vi "一台设备.vi"() -> ()   [LabVIEW 2012]
uses:
  <vilib>/Analysis/NI_AALPro.lvlib
panel:
  in  "?":enum32{"振动", "FFT", "转速", "温度湿度"}(tab)
  out "?":i16[](graph)
  out "?":i16[](graph)
  out "?":i16[](graph)
  out "?":i16[](graph)
  out "?":dbl[](graph)
  out "?":dbl[](graph)
  out "?":dbl[](graph)
  out "?":dbl[](graph)
  out "?":u16[](graph)
  out "?":dbl(graph)
  out "?":dbl(graph)
  out "?":dbl(graph)
  out "?":dbl(graph)
  out "?":dbl(graph)
  out "?":dbl(graph)
  out "?":u8(graph)
  out "?":u8(graph)
  out "系统时间":string
  out "收包":i32
  out "KB/s":dbl
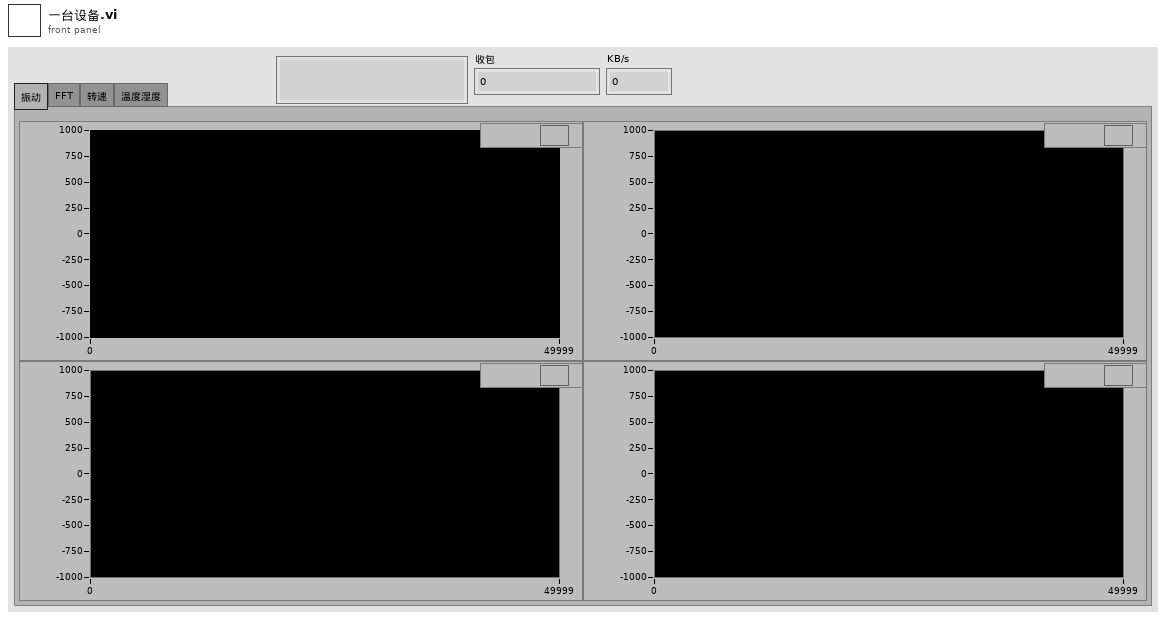
[diagram p1: front panel]
types:
  T1 = enum16{"open", "replace", "create", "open or create", "replace or create", "replace or create with confirmation"}
  T2 = enum16{"big-endian, network order", "native, host order", "little-endian"}
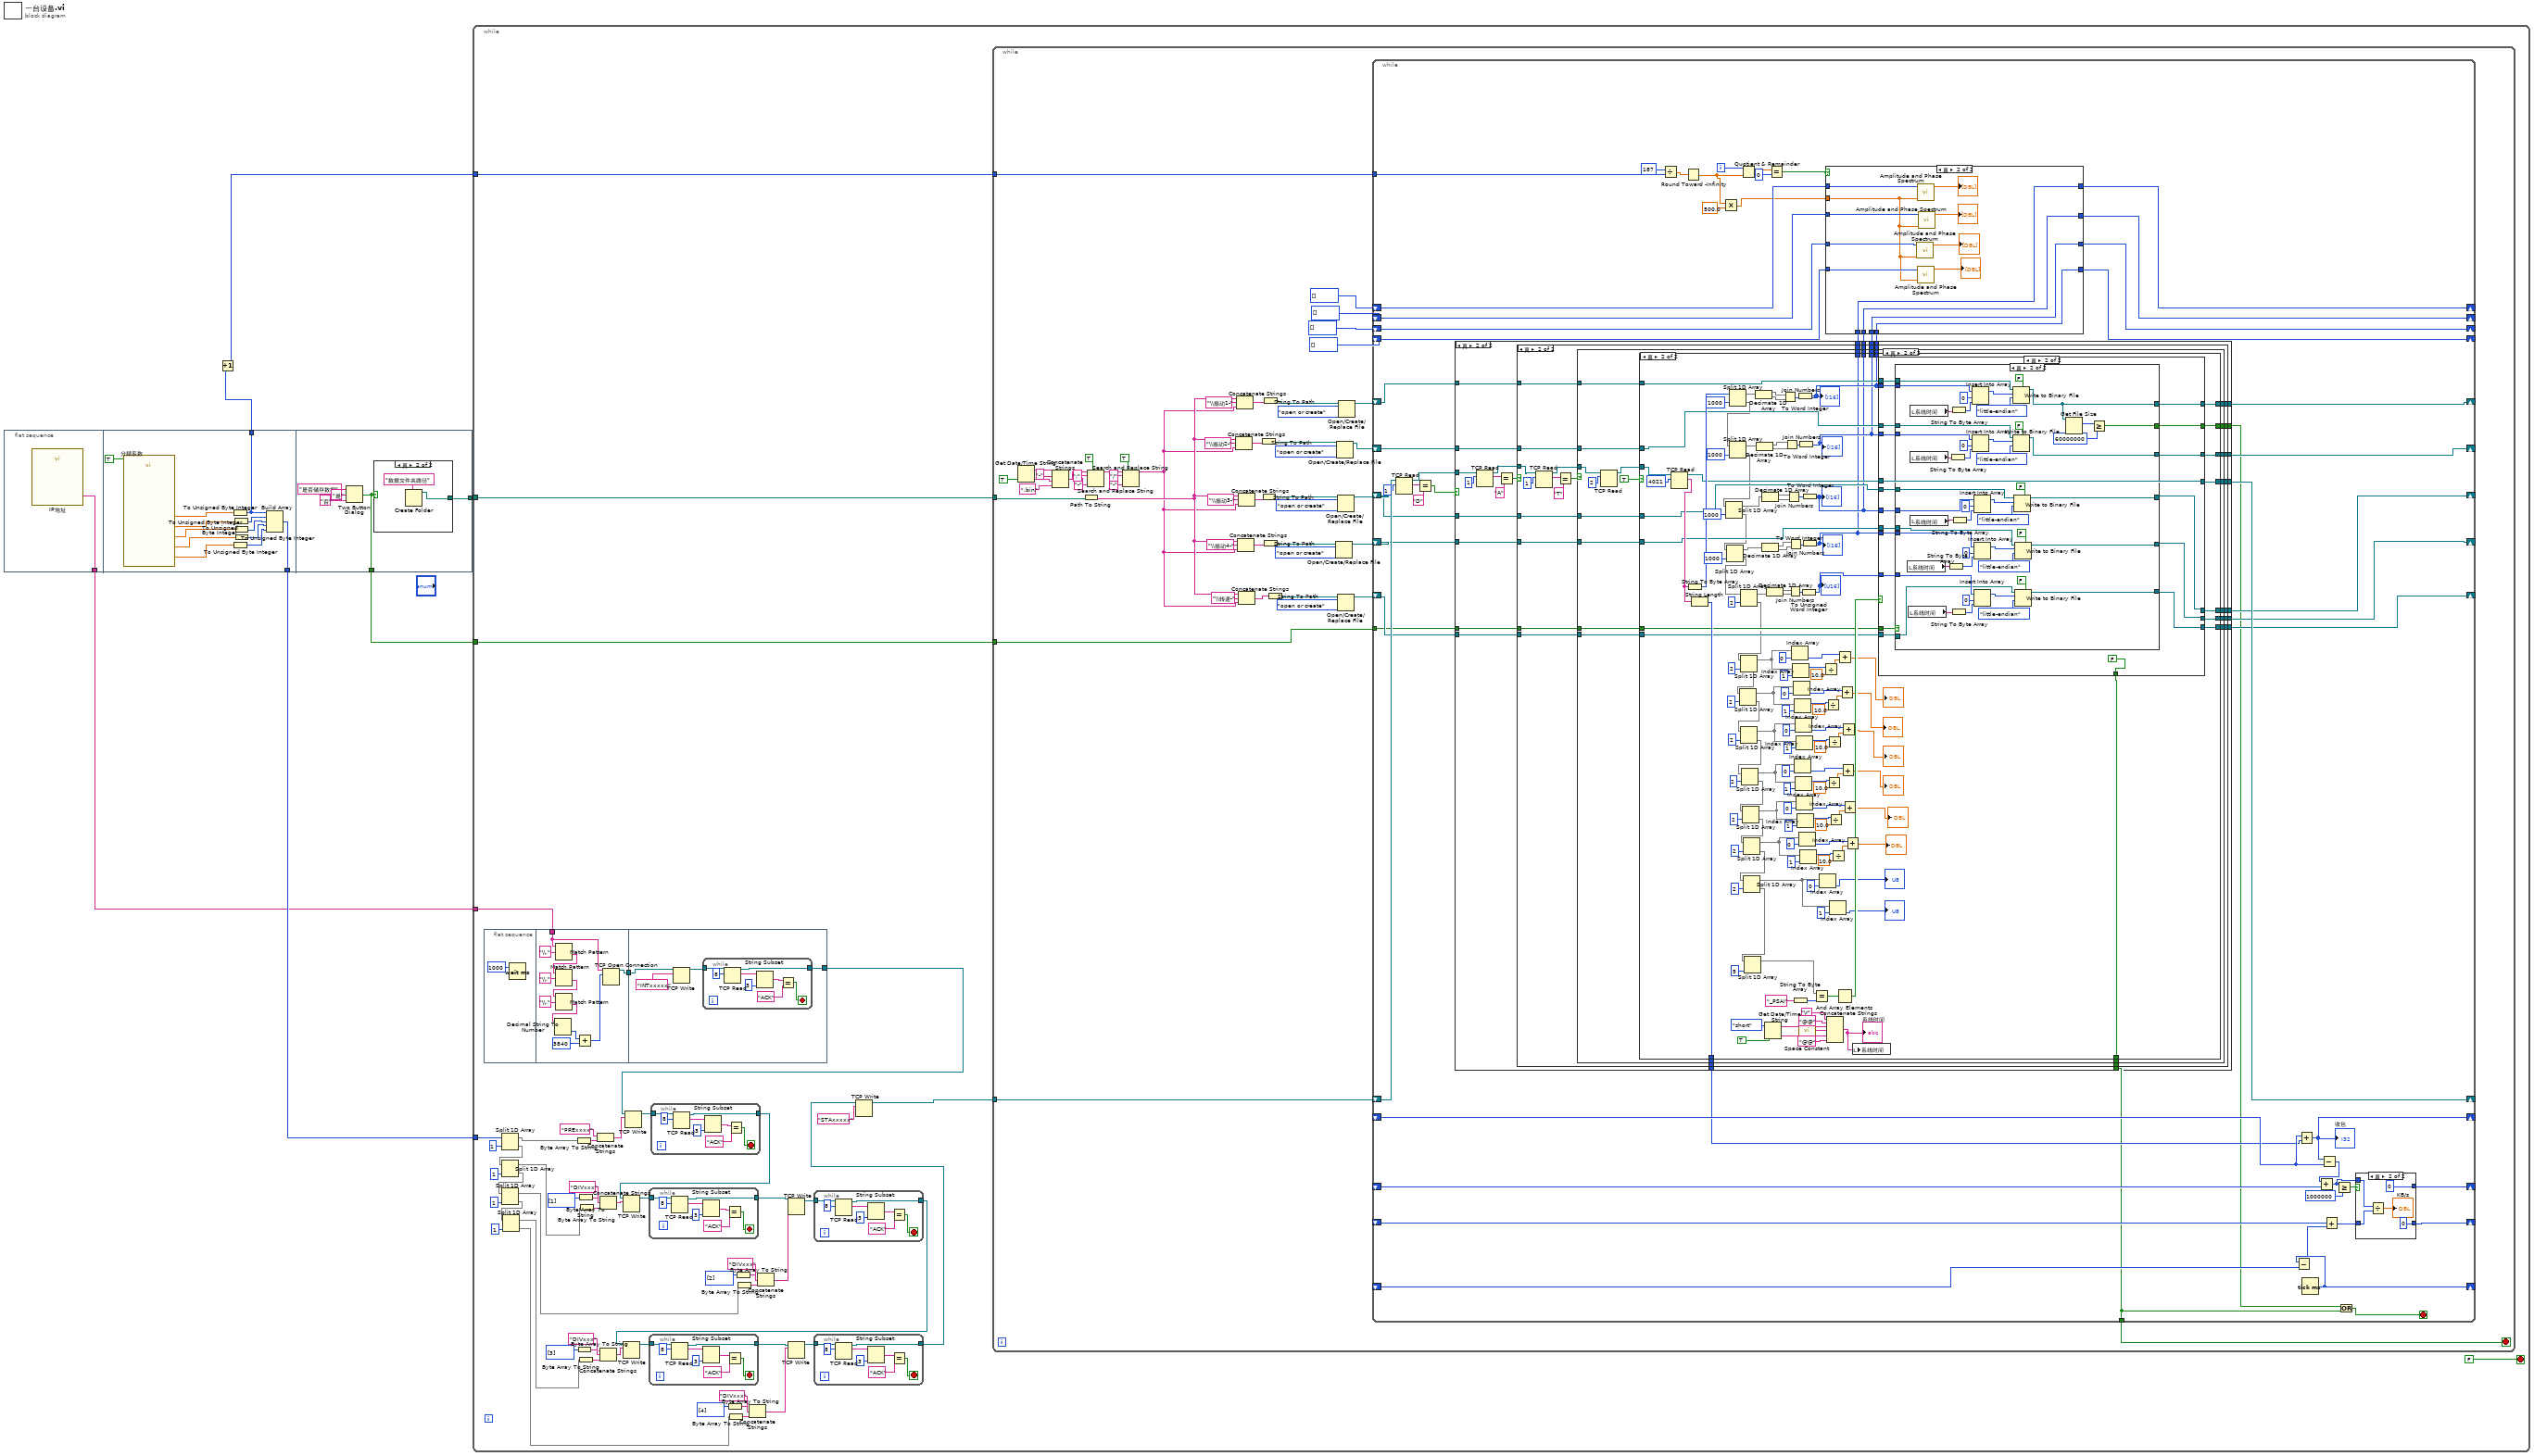
[diagram p0: block diagram]
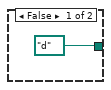
[diagram p2: hidden frame]
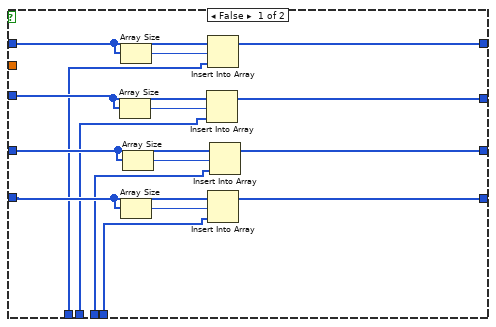
[diagram p3: hidden frame]
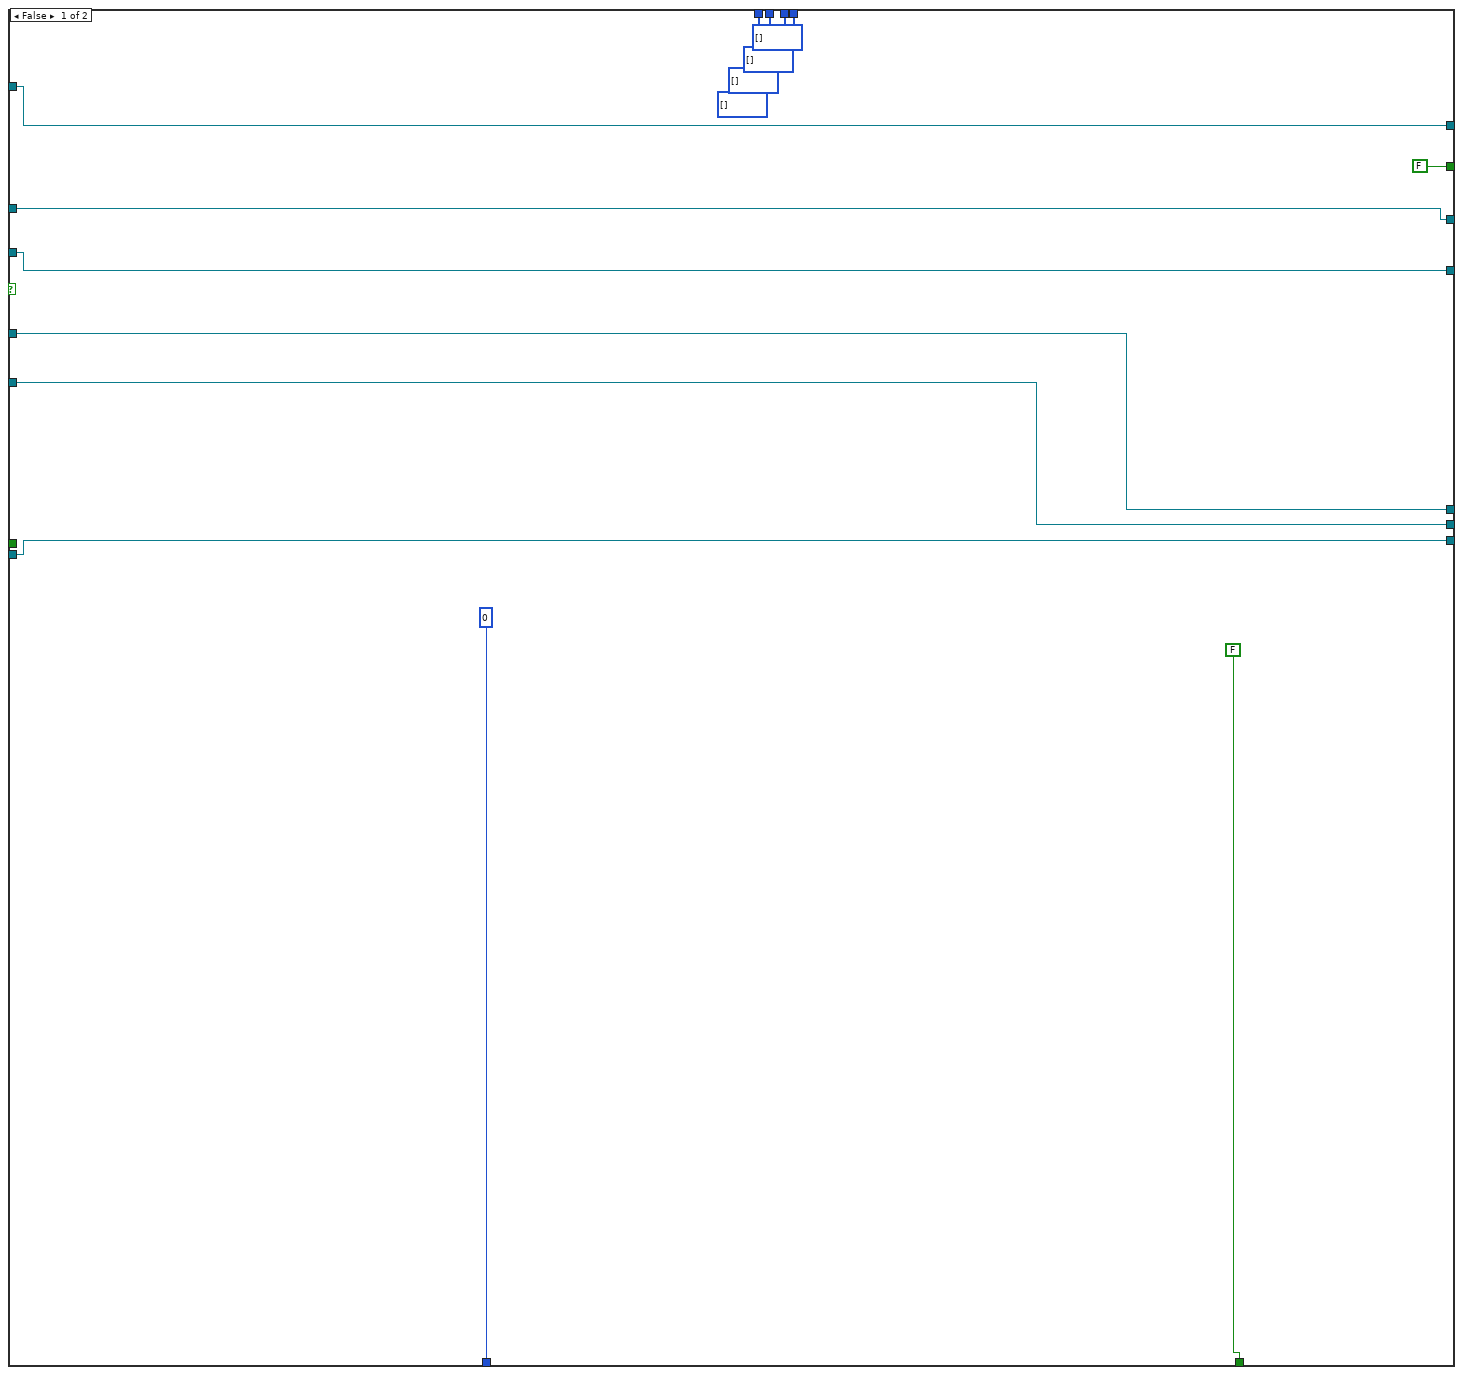
[diagram p4: hidden frame]
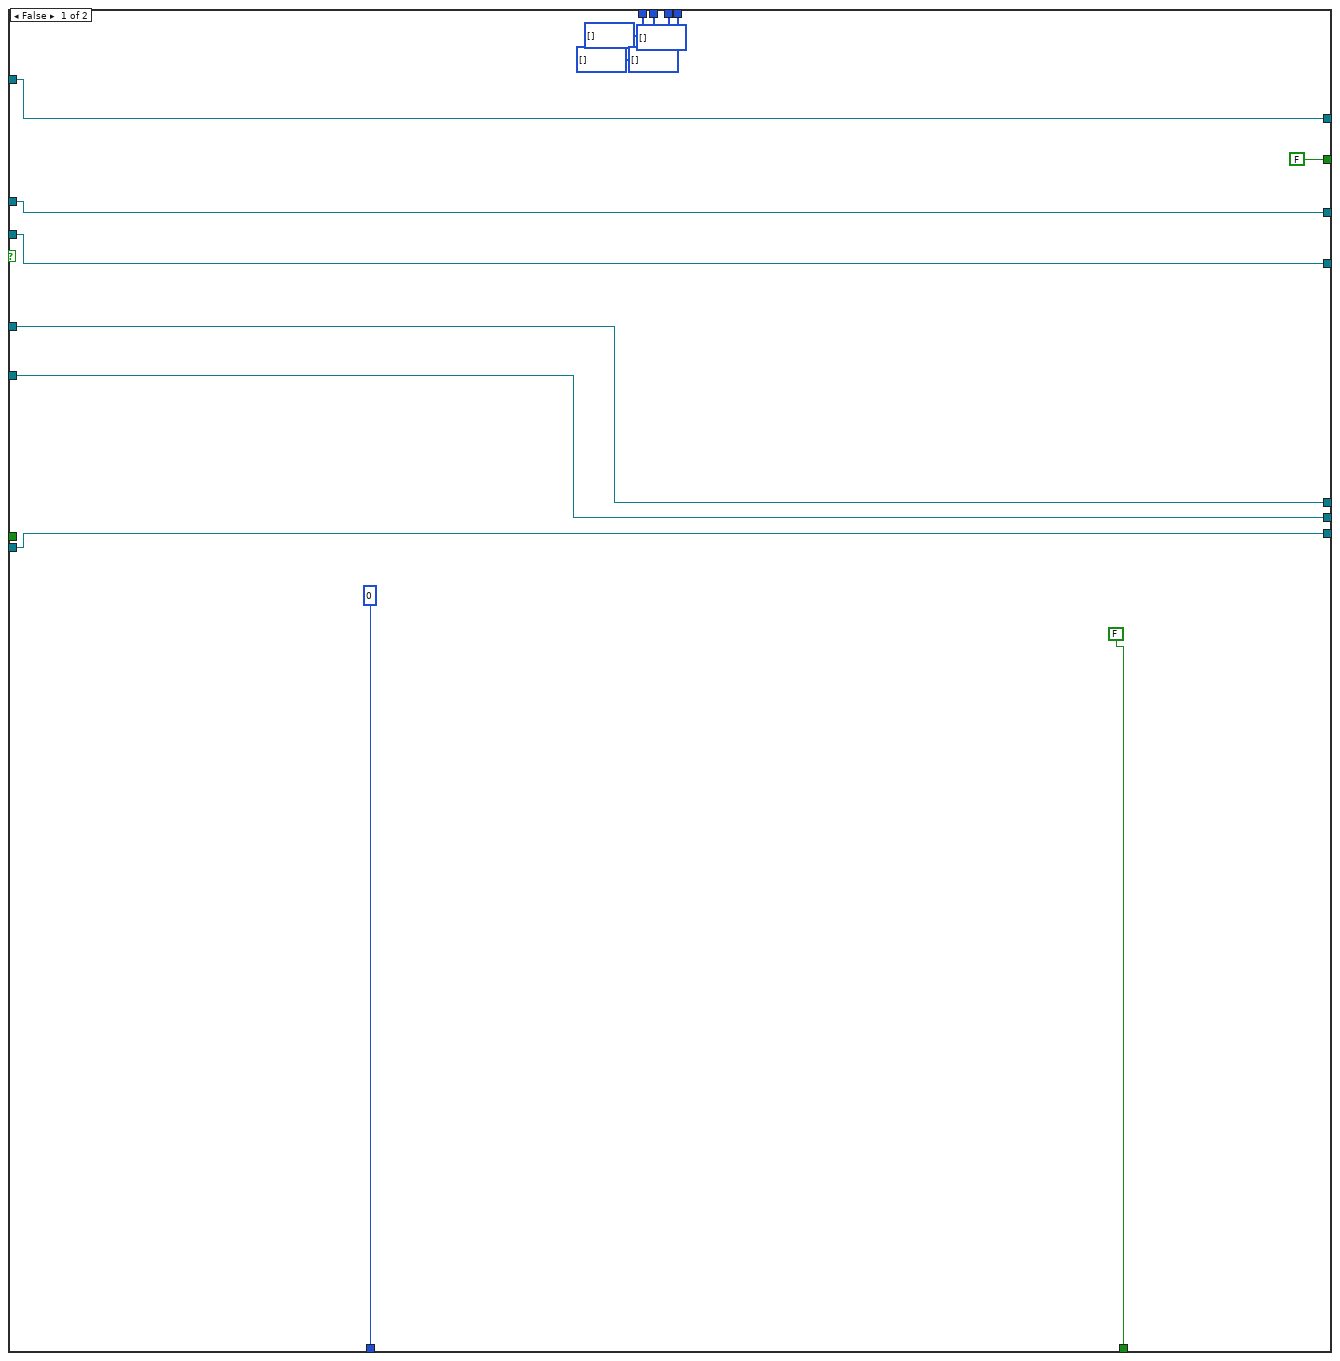
[diagram p5: hidden frame]
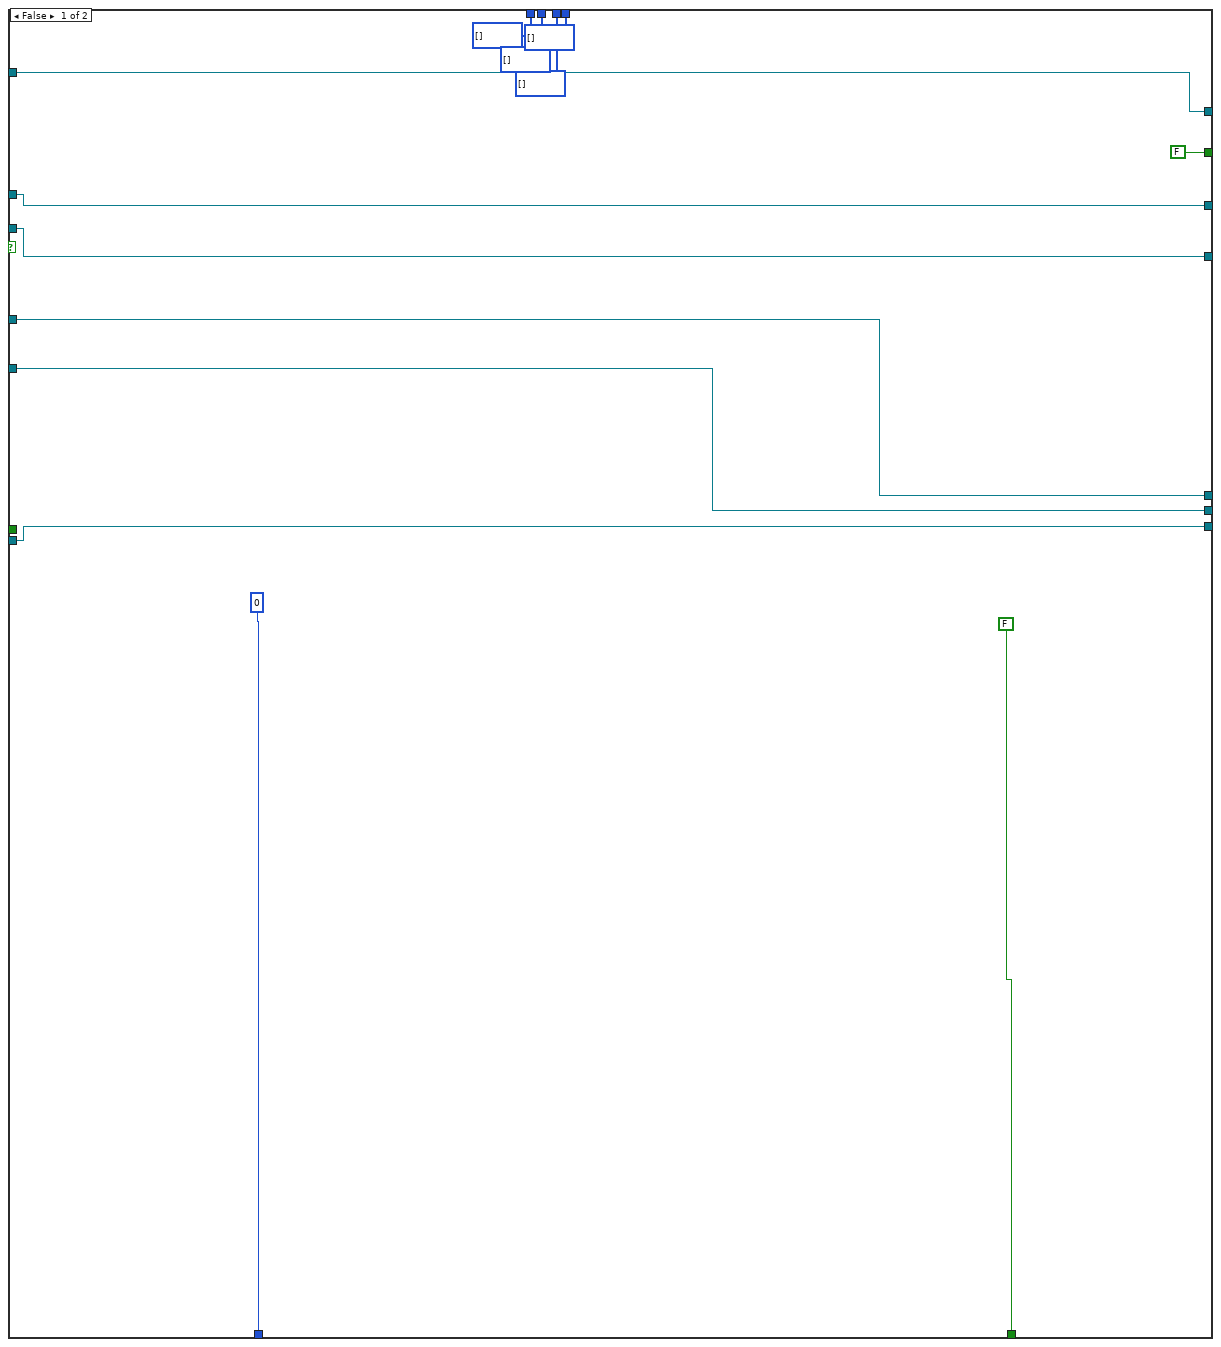
[diagram p6: hidden frame]
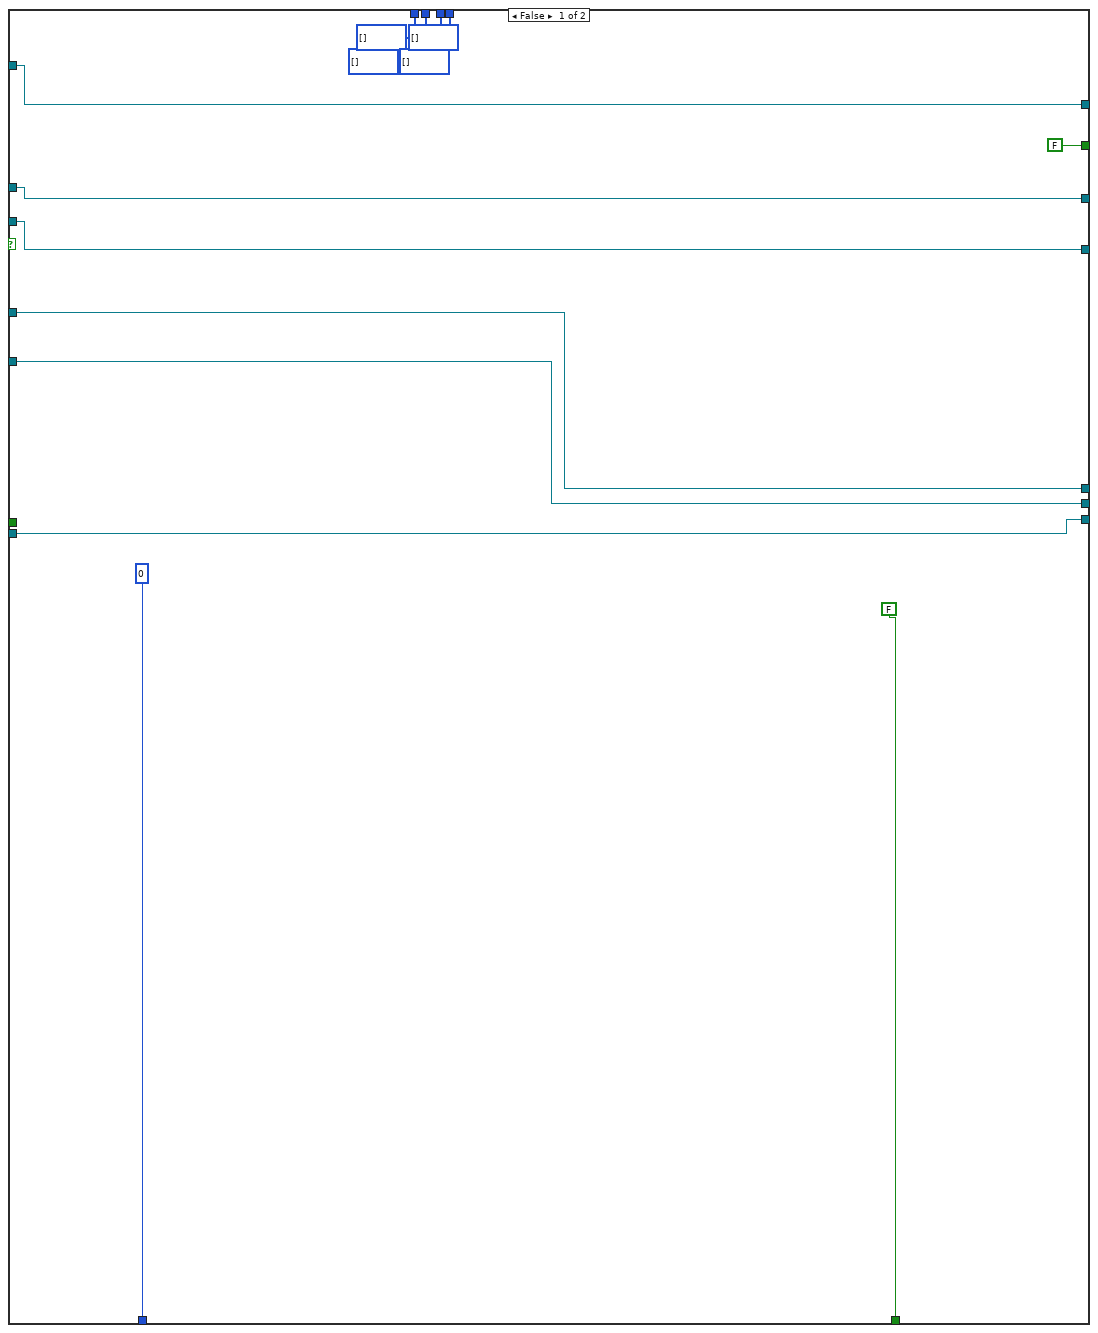
[diagram p7: hidden frame]
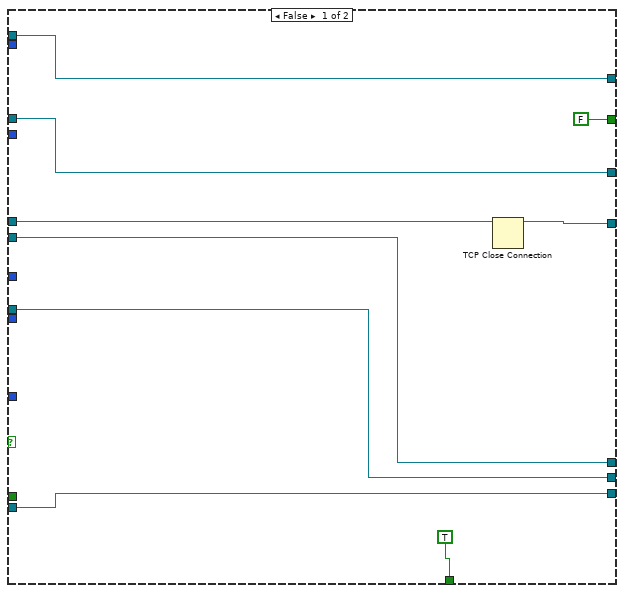
[diagram p8: hidden frame]
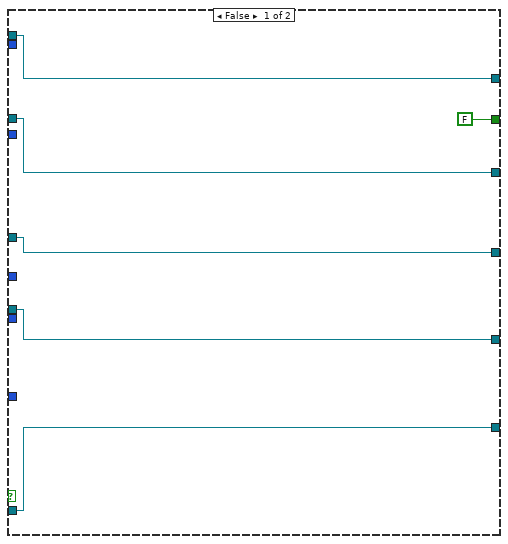
[diagram p9: hidden frame]
diagram:
  n1 = flat-sequence {
    tunnel: [w7] -> w1
    tunnel: [w14] -> w4
    tunnel: [w8] -> w3
    tunnel: [w21] -> w5
    tunnel: [w20] -> w6
    frame #0 {
      n2 = call "IP地址"() -> ("IP地址"=w7:string)  [unwired: 17 in, 2 out]
    }
    frame #1 {
      n3 = call "分频系数"("Enable"=TRUE) -> ("#4分频系数"=w12:dbl, "#3分频系数"=w11:dbl, "#2分频系数"=w10:dbl, "#1分频系数"=w9:dbl, "总分频系数"=w13:dbl)  [unwired: 12 in, 2 out]
      n4 = To Unsigned Byte Integer(number=w13) -> (unsigned 8bit integer=w8:u8)
      n5 = To Unsigned Byte Integer(number=w12) -> (unsigned 8bit integer=w15:u8)
      n6 = To Unsigned Byte Integer(number=w9) -> (unsigned 8bit integer=w18:u8)
      n7 = To Unsigned Byte Integer(number=w10) -> (unsigned 8bit integer=w17:u8)
      n8 = To Unsigned Byte Integer(number=w11) -> (unsigned 8bit integer=w16:u8)
      n9 = Build Array(w8, w18, w17, w16, w15) -> (w14:u8[])
    }
    frame #2 {
      n10 = Two Button Dialog(message="是否储存数据" ("消息"), 1:"否" ("F按钮名称（“取消”）"), 2:"是" ("T按钮名称（“确定”）")) -> (T button?=w20:bool)
      n11 = case shown="真" w20 {
        tunnel: [path "d:/" ("路径（使用对话框）") w27] -> w21
        frame False {
        }
        frame True {
          n12 = Create Folder(prompt (Create Folder)="数据文件夹路径" ("对话框窗口（创建文件夹）")) -> (created path=w27:path)  [unwired: 2 in, 2 out]
        }
      }
    }
  }
  n13 = Increment(x=w3) -> (x+1=w2:u8)
  n14 = while {
    tunnel: w6 -> [w81]
    tunnel: w5 -> [w80]
    tunnel: w4 -> [w66]
    tunnel: w2 -> [w79]
    tunnel: w1 -> [w28]
    stop <- FALSE stop-if-true
    n15 = flat-sequence {
      tunnel: [w94] -> w30
      tunnel: w28 -> [w85]
      tunnel: w30 -> [w97]
      tunnel: [w95] -> w29
      frame #0 {
        n16 = Wait (ms)(milliseconds to wait=u32 1000 ("毫秒倍数")) -> ()  [unwired: 1 out]
      }
      frame #1 {
        n17 = Match Pattern(string=w85, regular expression="\\." ("正则表达式")) -> (after substring=w89:string)  [unwired: 1 in, 3 out]
        n18 = Match Pattern(string=w89, regular expression="\\." ("正则表达式")) -> (after substring=w90:string)  [unwired: 1 in, 3 out]
        n19 = Match Pattern(string=w90, regular expression="\\." ("正则表达式")) -> (after substring=w91:string)  [unwired: 1 in, 3 out]
        n20 = Decimal String To Number(string=w91) -> (number=w92:i32)  [unwired: 2 in, 1 out]
        n21 = Add(x=w92, y=3840) -> (x+y=w84:i32)
        n22 = TCP Open Connection(address=w85, remote port or service name=w84) -> (connection ID=w94:refnum<k5>)  [unwired: 3 in, 1 out]
      }
      frame #2 {
        n23 = TCP Write(connection ID=w97, data in="INTxxxxx" ("数据输入")) -> (connection ID out=w96:refnum<k5>)  [unwired: 2 in, 2 out]
        n24 = while {
          tunnel: w96 -> [w106]
          tunnel: [w100] -> w95
          stop <- w101 stop-if-true
          n25 = TCP Read(connection ID=w106, bytes to read=8 ("读取的字节")) -> (connection ID out=w100:refnum<k5>, data out=w104:string)  [unwired: 3 in, 1 out]
          n26 = String Subset(string=w104, length (rest)=3 ("偏移量(0)")) -> (substring=w103:string)  [unwired: 1 in]
          n27 = Equal?(x=w103, y="ACK") -> (x = y?=w101:bool)
        }
      }
    }
    n28 = Split 1D Array(array=w66, index=1 ("索引")) -> (first subarray=w64:u8[], second subarray=w60:u8[])
    n29 = Split 1D Array(array=w60, index=1 ("索引")) -> (first subarray=w40:u8[], second subarray=w59:u8[])
    n30 = Split 1D Array(array=w59, index=1 ("索引")) -> (first subarray=w39:u8[], second subarray=w58:u8[])
    n31 = Split 1D Array(array=w58, index=1 ("索引")) -> (first subarray=w38:u8[], second subarray=w37:u8[])
    n32 = Byte Array To String(unsigned byte array=w64) -> (string=w69:string)
    n33 = Byte Array To String(unsigned byte array=u8[] [3] ("无符号字节数组")) -> (string=w46:string)
    n34 = Byte Array To String(unsigned byte array=u8[] [1] ("无符号字节数组")) -> (string=w54:string)
    n35 = Byte Array To String(unsigned byte array=w38) -> (string=w48:string)
    n36 = Byte Array To String(unsigned byte array=w40) -> (string=w57:string)
    n37 = Concatenate Strings("PRExxxx" ("数据输入"), w69) -> (w67:string)
    n38 = Concatenate Strings("DIVxxx" ("数据输入"), w54, w57) -> (w56:string)
    n39 = Concatenate Strings("DIVxxx" ("数据输入"), w46, w48) -> (w31:string)
    n40 = TCP Write(connection ID=w29, data in=w67) -> (connection ID out=w78:refnum<k5>)  [unwired: 2 in, 2 out]
    n41 = while {
      tunnel: w78 -> [w146]
      tunnel: [w140] -> w73
      stop <- w141 stop-if-true
      n42 = TCP Read(connection ID=w146, bytes to read=8 ("读取的字节")) -> (connection ID out=w140:refnum<k5>, data out=w144:string)  [unwired: 3 in, 1 out]
      n43 = String Subset(string=w144, length (rest)=3 ("偏移量(0)")) -> (substring=w143:string)  [unwired: 1 in]
      n44 = Equal?(x=w143, y="ACK") -> (x = y?=w141:bool)
    }
    n45 = TCP Write(connection ID=w73, data in=w56) -> (connection ID out=w77:refnum<k5>)  [unwired: 2 in, 2 out]
    n46 = while {
      tunnel: w77 -> [w138]
      tunnel: [w132] -> w72
      stop <- w133 stop-if-true
      n47 = TCP Read(connection ID=w138, bytes to read=8 ("读取的字节")) -> (connection ID out=w132:refnum<k5>, data out=w136:string)  [unwired: 3 in, 1 out]
      n48 = String Subset(string=w136, length (rest)=3 ("偏移量(0)")) -> (substring=w135:string)  [unwired: 1 in]
      n49 = Equal?(x=w135, y="ACK") -> (x = y?=w133:bool)
    }
    n50 = Byte Array To String(unsigned byte array=u8[] [4] ("无符号字节数组")) -> (string=w42:string)
    n51 = Byte Array To String(unsigned byte array=w37) -> (string=w44:string)
    n52 = Byte Array To String(unsigned byte array=u8[] [2] ("无符号字节数组")) -> (string=w50:string)
    n53 = Byte Array To String(unsigned byte array=w39) -> (string=w52:string)
    n54 = Concatenate Strings("DIVxxx" ("数据输入"), w42, w44) -> (w35:string)
    n55 = Concatenate Strings("DIVxxx" ("数据输入"), w50, w52) -> (w36:string)
    n56 = TCP Write(connection ID=w72, data in=w36) -> (connection ID out=w76:refnum<k5>)  [unwired: 2 in, 2 out]
    n57 = while {
      tunnel: w76 -> [w130]
      tunnel: [w124] -> w71
      stop <- w125 stop-if-true
      n58 = TCP Read(connection ID=w130, bytes to read=8 ("读取的字节")) -> (connection ID out=w124:refnum<k5>, data out=w128:string)  [unwired: 3 in, 1 out]
      n59 = String Subset(string=w128, length (rest)=3 ("偏移量(0)")) -> (substring=w127:string)  [unwired: 1 in]
      n60 = Equal?(x=w127, y="ACK") -> (x = y?=w125:bool)
    }
    n61 = TCP Write(connection ID=w71, data in=w31) -> (connection ID out=w75:refnum<k5>)  [unwired: 2 in, 2 out]
    n62 = while {
      tunnel: w75 -> [w122]
      tunnel: [w116] -> w70
      stop <- w117 stop-if-true
      n63 = TCP Read(connection ID=w122, bytes to read=8 ("读取的字节")) -> (connection ID out=w116:refnum<k5>, data out=w120:string)  [unwired: 3 in, 1 out]
      n64 = String Subset(string=w120, length (rest)=3 ("偏移量(0)")) -> (substring=w119:string)  [unwired: 1 in]
      n65 = Equal?(x=w119, y="ACK") -> (x = y?=w117:bool)
    }
    n66 = TCP Write(connection ID=w70, data in=w35) -> (connection ID out=w74:refnum<k5>)  [unwired: 2 in, 2 out]
    n67 = while {
      tunnel: w74 -> [w114]
      tunnel: [w108] -> w34
      stop <- w109 stop-if-true
      n68 = TCP Read(connection ID=w114, bytes to read=8 ("读取的字节")) -> (connection ID out=w108:refnum<k5>, data out=w112:string)  [unwired: 3 in, 1 out]
      n69 = String Subset(string=w112, length (rest)=3 ("偏移量(0)")) -> (substring=w111:string)  [unwired: 1 in]
      n70 = Equal?(x=w111, y="ACK") -> (x = y?=w109:bool)
    }
    n71 = TCP Write(connection ID=w34, data in="STAxxxxx" ("数据输入")) -> (connection ID out=w32:refnum<k5>)  [unwired: 2 in, 2 out]
    n72 = while {
      tunnel: w32 -> [w195]
      tunnel: w81 -> [w194]
      tunnel: w80 -> [w167]
      tunnel: w79 -> [w147]
      stop <- w157 stop-if-true
      n73 = Get Date/Time String(want seconds? (F)=TRUE ("需要秒？(F)")) -> (date string=w165:string, time string=w162:string)  [unwired: 2 in]
      n74 = Concatenate Strings(w165, "-" ("字符串"), w162, ".bin" ("字符串")) -> (w161:string)
      n75 = Path To String(path=w167) -> (string=w178:string)
      n76 = Search and Replace String(replace all?=TRUE ("替换全部？(F)"), input string=w161, search string=":" ("搜索字符串"), replace string="-" ("替换字符串(\"\")")) -> (result string=w153:string)  [unwired: 4 in, 3 out]
      n77 = Search and Replace String(replace all?=TRUE ("替换全部？(F)"), input string=w153, search string="/" ("搜索字符串"), replace string="-" ("替换字符串(\"\")")) -> (result string=w152:string)  [unwired: 4 in, 3 out]
      n78 = Concatenate Strings(w178, "\\振动2-" ("字符串"), w152) -> (w185:string)
      n79 = Concatenate Strings(w178, "\\振动1-" ("字符串"), w152) -> (w184:string)
      n80 = Concatenate Strings(w178, "\\振动4-" ("字符串"), w152) -> (w187:string)
      n81 = Concatenate Strings(w178, "\\振动3-" ("字符串"), w152) -> (w186:string)
      n82 = Concatenate Strings(w178, "\\转速-" ("字符串"), w152) -> (w188:string)
      n83 = String To Path(string=w185) -> (path=w182:path)
      n84 = String To Path(string=w186) -> (path=w181:path)
      n85 = String To Path(string=w184) -> (path=w183:path)
      n86 = String To Path(string=w187) -> (path=w180:path)
      n87 = String To Path(string=w188) -> (path=w179:path)
      n88 = Open/Create/Replace File(file path (use dialog)=w180, operation (0:open)=T1."open or create" ("操作(0:open)")) -> (refnum out=w169:refnum<file>)  [unwired: 4 in, 2 out]
      n89 = Open/Create/Replace File(file path (use dialog)=w182, operation (0:open)=T1."open or create" ("操作(0:open)")) -> (refnum out=w171:refnum<file>)  [unwired: 4 in, 2 out]
      n90 = Open/Create/Replace File(file path (use dialog)=w181, operation (0:open)=T1."open or create" ("操作(0:open)")) -> (refnum out=w170:refnum<file>)  [unwired: 4 in, 2 out]
      n91 = Open/Create/Replace File(file path (use dialog)=w179, operation (0:open)=T1."open or create" ("操作(0:open)")) -> (refnum out=w168:refnum<file>)  [unwired: 4 in, 2 out]
      n92 = Open/Create/Replace File(file path (use dialog)=w183, operation (0:open)=T1."open or create" ("操作(0:open)")) -> (refnum out=w172:refnum<file>)  [unwired: 4 in, 2 out]
      n93 = while {
        shift-right: [w253] -> _
        shift-left: _ -> [w252]
        shift-right: [w235] -> _
        shift-left: w195 -> [w239]
        shift-right: [w247] -> _
        shift-left: _ -> [w250]
        shift-right: [w244] -> _
        shift-left: _ -> [w245]
        shift-right: [w242] -> _
        shift-left: _ -> [w240]
        shift-right: [w231] -> _
        shift-left: w172 -> [w226]
        shift-right: [w230] -> _
        shift-left: w171 -> [w225]
        shift-right: [w229] -> _
        shift-left: w170 -> [w224]
        shift-right: [w228] -> _
        shift-left: w169 -> [w223]
        shift-right: [w227] -> _
        shift-left: w168 -> [w222]
        tunnel: w194 -> [w221]
        tunnel: [w219] -> w157
        shift-right: [w203] -> _
        shift-left: i16[] [] -> [w207]
        shift-right: [w204] -> _
        shift-left: i16[] [] -> [w208]
        shift-right: [w205] -> _
        shift-left: i16[] [] -> [w209]
        shift-right: [w206] -> _
        shift-left: i16[] [] -> [w202]
        tunnel: w147 -> [w198]
        i -> [w217]
        stop <- w218 stop-if-true
        n94 = TCP Read(connection ID=w239, bytes to read=1 ("读取的字节")) -> (connection ID out=w232:refnum<k5>, data out=w237:string)  [unwired: 3 in, 1 out]
        n95 = Equal?(x=w237, y="D") -> (x = y?=w233:bool)
        n96 = case shown="真" w233 {
          tunnel: w232 -> [w295 w316]
          tunnel: [w295 w315] -> w235
          tunnel: [0 w314] -> w234
          tunnel: [FALSE w312] -> w219
          tunnel: [w292 w311] -> w231
          tunnel: [w291 w304] -> w230
          tunnel: [w290 w303] -> w229
          tunnel: [w289 w302] -> w228
          tunnel: [w288 w310] -> w227
          tunnel: w226 -> [w292 w309]
          tunnel: w225 -> [w291 w308]
          tunnel: w224 -> [w290 w307]
          tunnel: w223 -> [w289 w306]
          tunnel: w222 -> [w288 w305]
          tunnel: w221 -> [_ w301]
          tunnel: [FALSE w300] -> w220
          tunnel: [i16[] [] w299] -> w213
          tunnel: [i16[] [] w298] -> w212
          tunnel: [i16[] [] w297] -> w211
          tunnel: [i16[] [] w296] -> w210
          frame False {
          }
          frame True {
            n97 = TCP Read(connection ID=w316, bytes to read=1 ("读取的字节")) -> (connection ID out=w313:refnum<k5>, data out=w319:string)  [unwired: 3 in, 1 out]
            n98 = Equal?(x=w319, y="A") -> (x = y?=w317:bool)
            n99 = case shown="真" w317 {
              tunnel: w313 -> [w333 w354]
              tunnel: [w333 w353] -> w315
              tunnel: [0 w352] -> w314
              tunnel: [FALSE w350] -> w312
              tunnel: [w330 w349] -> w311
              tunnel: [w326 w345] -> w310
              tunnel: w309 -> [w330 w344]
              tunnel: w308 -> [w329 w343]
              tunnel: w307 -> [w328 w342]
              tunnel: w306 -> [w327 w341]
              tunnel: w305 -> [w326 w340]
              tunnel: [w329 w348] -> w304
              tunnel: [w328 w347] -> w303
              tunnel: [w327 w346] -> w302
              tunnel: w301 -> [_ w339]
              tunnel: [FALSE w338] -> w300
              tunnel: [i16[] [] w337] -> w299
              tunnel: [i16[] [] w336] -> w298
              tunnel: [i16[] [] w335] -> w297
              tunnel: [i16[] [] w334] -> w296
              frame False {
              }
              frame True {
                n100 = TCP Read(connection ID=w354, bytes to read=1 ("读取的字节")) -> (connection ID out=w351:refnum<k5>, data out=w357:string)  [unwired: 3 in, 1 out]
                n101 = Equal?(x=w357, y="T") -> (x = y?=w355:bool)
                n102 = case shown="真" w355 {
                  tunnel: w351 -> [w371 w393]
                  tunnel: [w371 w390] -> w353
                  tunnel: [0 w392] -> w352
                  tunnel: [FALSE w389] -> w350
                  tunnel: [w364 w381] -> w349
                  tunnel: [w365 w380] -> w348
                  tunnel: [w366 w379] -> w347
                  tunnel: [w367 w388] -> w346
                  tunnel: [w368 w387] -> w345
                  tunnel: w344 -> [w364 w386]
                  tunnel: w343 -> [w365 w385]
                  tunnel: w342 -> [w366 w384]
                  tunnel: w341 -> [w367 w383]
                  tunnel: w340 -> [w368 w382]
                  tunnel: w339 -> [_ w378]
                  tunnel: [FALSE w377] -> w338
                  tunnel: [i16[] [] w376] -> w337
                  tunnel: [i16[] [] w375] -> w336
                  tunnel: [i16[] [] w374] -> w335
                  tunnel: [i16[] [] w373] -> w334
                  frame False {
                  }
                  frame True {
                    n103 = TCP Read(connection ID=w393, bytes to read=2 ("读取的字节")) -> (connection ID out=w391:refnum<k5>)  [unwired: 3 in, 2 out]
                    n104 = case shown="真" TRUE {
                      tunnel: w391 -> [w407 w543]
                      tunnel: [0 w534] -> w392
                      tunnel: [w407 w527] -> w390
                      tunnel: [FALSE w528] -> w389
                      tunnel: [w401 w510] -> w388
                      tunnel: [w400 w509] -> w387
                      tunnel: w386 -> [w404 w516]
                      tunnel: w385 -> [w403 w514]
                      tunnel: w384 -> [w402 w512]
                      tunnel: w383 -> [w401 w436]
                      tunnel: w382 -> [w400 w508]
                      tunnel: [w404 w515] -> w381
                      tunnel: [w403 w513] -> w380
                      tunnel: [w402 w511] -> w379
                      tunnel: w378 -> [_ w506]
                      tunnel: [FALSE w504] -> w377
                      tunnel: [i16[] [] w435] -> w376
                      tunnel: [i16[] [] w434] -> w375
                      tunnel: [i16[] [] w433] -> w374
                      tunnel: [i16[] [] w432] -> w373
                      frame False {
                      }
                      frame True {
                        n105 = TCP Read(connection ID=w543, bytes to read=4021 ("最大值(548)")) -> (connection ID out=w517:refnum<k5>, data out=w526:string)  [unwired: 3 in, 1 out]
                        n106 = String To Byte Array(string=w526) -> (unsigned byte array=w525:u8[])
                        n107 = String Length(string=w526) -> (length=w534:i32)
                        n108 = Split 1D Array(array=w525, index=1000 ("索引")) -> (first subarray=w430:u8[], second subarray=w427:u8[])
                        n109 = Split 1D Array(array=w427, index=1000 ("索引")) -> (first subarray=w426:u8[], second subarray=w423:u8[])
                        n110 = Split 1D Array(array=w423, index=1000 ("索引")) -> (first subarray=w422:u8[], second subarray=w421:u8[])
                        n111 = Split 1D Array(array=w421, index=1000 ("索引")) -> (first subarray=w418:u8[], second subarray=w431:u8[])
                        n112 = Split 1D Array(array=w431, index=2 ("索引")) -> (first subarray=w415:u8[], second subarray=w503:u8[])
                        n113 = Split 1D Array(array=w503, index=2 ("索引")) -> (first subarray=w486:u8[], second subarray=w502:u8[])
                        n114 = Split 1D Array(array=w502, index=2 ("索引")) -> (first subarray=w450:u8[], second subarray=w501:u8[])
                        n115 = Split 1D Array(array=w501, index=2 ("索引")) -> (first subarray=w449:u8[], second subarray=w488:u8[])
                        n116 = Split 1D Array(array=w488, index=2 ("索引")) -> (first subarray=w448:u8[], second subarray=w497:u8[])
                        n117 = Split 1D Array(array=w497, index=2 ("索引")) -> (first subarray=w447:u8[], second subarray=w496:u8[])
                        n118 = Split 1D Array(array=w496, index=2 ("索引")) -> (first subarray=w446:u8[], second subarray=w487:u8[])
                        n119 = Split 1D Array(array=w487, index=2 ("索引")) -> (first subarray=w445:u8[], second subarray=w409:u8[])
                        n120 = Split 1D Array(array=w409, index=5 ("索引")) -> (first subarray=w408:u8[])  [unwired: 1 out]
                        n121 = Decimate 1D Array(w430) -> (w429:u8[], w428:u8[])
                        n122 = Decimate 1D Array(w426) -> (w425:u8[], w424:u8[])
                        n123 = Decimate 1D Array(w422) -> (w420:u8[], w419:u8[])
                        n124 = Decimate 1D Array(w418) -> (w417:u8[], w416:u8[])
                        n125 = Get Date/Time String(date format (0)=enum16{"short", "long", "abbreviated"}."short" ("日期格式(0)"), want seconds? (F)=TRUE ("需要秒？(F)")) -> (date string=w522:string, time string=w505:string)  [unwired: 1 in]
                        n126 = Decimate 1D Array(w415) -> (w414:u8[], w413:u8[])
                        n127 = Join Numbers(hi=w429, lo=w428) -> ((hi.lo)=w541:u16[])
                        n128 = Join Numbers(hi=w425, lo=w424) -> ((hi.lo)=w536:u16[])
                        n129 = Join Numbers(hi=w420, lo=w419) -> ((hi.lo)=w537:u16[])
                        n130 = Join Numbers(hi=w414, lo=w413) -> ((hi.lo)=w411:u16[])
                        n131 = Join Numbers(hi=w417, lo=w416) -> ((hi.lo)=w538:u16[])
                        n132 = Index Array(array=w486, index=0 ("索引")) -> (element=w481:u8)
                        n133 = Index Array(array=w486, index=1 ("索引")) -> (element=w483:u8)
                        n134 = String To Byte Array(string="_PSAI") -> (unsigned byte array=w531:u8[])
                        n135 = Index Array(array=w450, index=0 ("索引")) -> (element=w475:u8)
                        n136 = Index Array(array=w450, index=1 ("索引")) -> (element=w477:u8)
                        n137 = Index Array(array=w448, index=0 ("索引")) -> (element=w463:u8)
                        n138 = Index Array(array=w449, index=0 ("索引")) -> (element=w469:u8)
                        n139 = Index Array(array=w448, index=1 ("索引")) -> (element=w465:u8)
                        n140 = Index Array(array=w449, index=1 ("索引")) -> (element=w471:u8)
                        n141 = Index Array(array=w447, index=0 ("索引")) -> (element=w457:u8)
                        n142 = To Word Integer(number=w541) -> (16bit integer=w435:i16[])
                        "?" <- w435
                        n143 = Index Array(array=w447, index=1 ("索引")) -> (element=w459:u8)
                        n144 = To Word Integer(number=w536) -> (16bit integer=w434:i16[])
                        "?" <- w434
                        n145 = Index Array(array=w446, index=0 ("索引")) -> (element=w451:u8)
                        n146 = call <vilib>:"Space Constant.vi"() -> ("String"=w518:string)
                        n147 = Index Array(array=w446, index=1 ("索引")) -> (element=w453:u8)
                        n148 = To Unsigned Word Integer(number=w411) -> (unsigned 16bit integer=w412:u16[])
                        "?" <- w412
                        n149 = To Word Integer(number=w537) -> (16bit integer=w433:i16[])
                        "?" <- w433
                        n150 = To Word Integer(number=w538) -> (16bit integer=w432:i16[])
                        "?" <- w432
                        n151 = Equal?(x=w408, y=w531) -> (x = y?=w530:bool[])
                        n152 = Index Array(array=w445, index=0 ("索引")) -> (element=→"?":u8)
                        n153 = Divide(x=w483, y=10.0) -> (x/y=w482:dbl)
                        n154 = Divide(x=w477, y=10.0) -> (x/y=w476:dbl)
                        n155 = Divide(x=w465, y=10.0) -> (x/y=w464:dbl)
                        n156 = Divide(x=w471, y=10.0) -> (x/y=w470:dbl)
                        n157 = Concatenate Strings("\r", "@@" ("字符串"), w522, w518, w505, "@@" ("字符串")) -> (w521:string)
                        "系统时间" <- w521
                        n158 = Divide(x=w459, y=10.0) -> (x/y=w458:dbl)
                        n159 = Index Array(array=w445, index=1 ("索引")) -> (element=→"?":u8)
                        n160 = Divide(x=w453, y=10.0) -> (x/y=w452:dbl)
                        n161 = And Array Elements(Boolean array=w530) -> (logical AND=w529:bool)
                        n162 = Add(x=w481, y=w482) -> (x+y=→"?":dbl)
                        n163 = Add(x=w475, y=w476) -> (x+y=→"?":dbl)
                        n164 = Add(x=w463, y=w464) -> (x+y=→"?":dbl)
                        n165 = Add(x=w469, y=w470) -> (x+y=→"?":dbl)
                        n166 = Add(x=w457, y=w458) -> (x+y=→"?":dbl)
                        n167 = Add(x=w451, y=w452) -> (x+y=→"?":dbl)
                        n168 = local write "系统时间"(w521) -> ()
                        n169 = case shown="真" w529 {
                          tunnel: [w553 w572] -> w527
                          tunnel: [TRUE FALSE] -> w528
                          tunnel: w517 -> [w551 w572]
                          tunnel: w435 -> [_ w571]
                          tunnel: w434 -> [_ w570]
                          tunnel: w433 -> [_ w569]
                          tunnel: w432 -> [_ w568]
                          tunnel: w412 -> [_ w567]
                          tunnel: w516 -> [w549 w565]
                          tunnel: [w549 w564] -> w515
                          tunnel: w514 -> [w550 w563]
                          tunnel: [w550 w562] -> w513
                          tunnel: w512 -> [w548 w561]
                          tunnel: [w548 w560] -> w511
                          tunnel: w436 -> [w547 w559]
                          tunnel: [w547 w558] -> w510
                          tunnel: [w546 w557] -> w509
                          tunnel: w508 -> [w546 w556]
                          tunnel: w506 -> [_ w555]
                          tunnel: [FALSE w554] -> w504
                          frame False {
                            n170 = TCP Close Connection(connection ID=w551) -> (connection ID out=w553:refnum<k5>)  [unwired: 2 in, 1 out]
                          }
                          frame True {
                            n171 = case shown="真" w555 {
                              tunnel: w571 -> [_ w625]
                              tunnel: w570 -> [_ w605]
                              tunnel: w569 -> [_ w604]
                              tunnel: w568 -> [_ w603]
                              tunnel: w567 -> [_ w602]
                              tunnel: w565 -> [w578 w591]
                              tunnel: [w578 w582] -> w564
                              tunnel: w563 -> [w577 w590]
                              tunnel: [w577 w589] -> w562
                              tunnel: w561 -> [w576 w588]
                              tunnel: [w576 w583] -> w560
                              tunnel: w559 -> [w575 w587]
                              tunnel: [w575 w586] -> w558
                              tunnel: [w574 w585] -> w557
                              tunnel: w556 -> [w574 w584]
                              tunnel: [FALSE w579] -> w554
                              frame False {
                              }
                              frame True {
                                n172 = local read "系统时间"() -> (w599:string)
                                n173 = local read "系统时间"() -> (w601:string)
                                n174 = local read "系统时间"() -> (w593:string)
                                n175 = local read "系统时间"() -> (w595:string)
                                n176 = local read "系统时间"() -> (w597:string)
                                n177 = String To Byte Array(string=w599) -> (unsigned byte array=w598:u8[])
                                n178 = String To Byte Array(string=w595) -> (unsigned byte array=w594:u8[])
                                n179 = String To Byte Array(string=w593) -> (unsigned byte array=w592:u8[])
                                n180 = String To Byte Array(string=w601) -> (unsigned byte array=w600:u8[])
                                n181 = String To Byte Array(string=w597) -> (unsigned byte array=w596:u8[])
                                n182 = Insert Into Array(array=w625, index=0 ("索引"), new element=w592) -> (w623:i16[])
                                n183 = Insert Into Array(array=w605, index=0 ("索引"), new element=w594) -> (w619:i16[])
                                n184 = Insert Into Array(array=w604, index=0 ("索引"), new element=w596) -> (w615:i16[])
                                n185 = Insert Into Array(array=w603, index=0 ("索引"), new element=w598) -> (w611:i16[])
                                n186 = Insert Into Array(array=w602, index=0 ("索引"), new element=w600) -> (w607:u16[])
                                n187 = Write to Binary File(file (use dialog)=w591, data=w623, 5:FALSE ("预置数组或字符串大小？(T)"), 9:T2."little-endian" ("字节顺序(0:big-endian, network order)")) -> (refnum out=w582:refnum<file>)  [unwired: 2 in, 2 out]
                                n188 = Write to Binary File(file (use dialog)=w590, data=w619, 5:FALSE ("预置数组或字符串大小？(T)"), 9:T2."little-endian" ("字节顺序(0:big-endian, network order)")) -> (refnum out=w589:refnum<file>)  [unwired: 2 in, 2 out]
                                n189 = Write to Binary File(file (use dialog)=w588, data=w615, 5:FALSE ("预置数组或字符串大小？(T)"), 9:T2."little-endian" ("字节顺序(0:big-endian, network order)")) -> (refnum out=w583:refnum<file>)  [unwired: 2 in, 2 out]
                                n190 = Write to Binary File(file (use dialog)=w587, data=w611, 5:FALSE ("预置数组或字符串大小？(T)"), 9:T2."little-endian" ("字节顺序(0:big-endian, network order)")) -> (refnum out=w586:refnum<file>)  [unwired: 2 in, 2 out]
                                n191 = Write to Binary File(file (use dialog)=w584, data=w607, 5:FALSE ("预置数组或字符串大小？(T)"), 9:T2."little-endian" ("字节顺序(0:big-endian, network order)")) -> (refnum out=w585:refnum<file>)  [unwired: 2 in, 2 out]
                                n192 = Get File Size(file=w582) -> (size (in bytes)=w581:i64)  [unwired: 1 in, 2 out]
                                n193 = Greater Or Equal?(x=w581, y=i64 60000000) -> (x >= y?=w579:bool)
                              }
                            }
                          }
                        }
                      }
                    }
                  }
                }
              }
            }
          }
        }
        n194 = Divide(x=u8 187, y=w198) -> (x/y=w196:dbl)
        n195 = Round Toward -Infinity(1:w196) -> (0:w200:dbl)
        n196 = Multiply(x=w200, y=500.0) -> (x*y=w199:dbl)
        n197 = Quotient & Remainder(x=w217, y=w200) -> (x-y*floor(x/y)=w216:dbl)  [unwired: 1 out]
        n198 = Equal?(x=w216, y=0) -> (x = y?=w214:bool)
        n199 = case shown="真" w214 {
          tunnel: w213 -> [w257 w282]
          tunnel: w212 -> [w256 w281]
          tunnel: w211 -> [w255 w280]
          tunnel: w210 -> [w254 w279]
          tunnel: [w265 w282] -> w203
          tunnel: [w264 w281] -> w204
          tunnel: [w263 w280] -> w205
          tunnel: [w262 w279] -> w206
          tunnel: w202 -> [w261 w275]
          tunnel: w209 -> [w260 w278]
          tunnel: w208 -> [w259 w276]
          tunnel: w207 -> [w258 w277]
          tunnel: w199 -> [_ w270]
          frame False {
            n200 = Array Size(array=w260) -> (size(s)=w267:i32)
            n201 = Array Size(array=w261) -> (size(s)=w266:i32)
            n202 = Array Size(array=w258) -> (size(s)=w269:i32)
            n203 = Array Size(array=w259) -> (size(s)=w268:i32)
            n204 = Insert Into Array(array=w260, index=w267, new element=w255) -> (w263:i16[])
            n205 = Insert Into Array(array=w261, index=w266, new element=w254) -> (w262:i16[])
            n206 = Insert Into Array(array=w258, index=w269, new element=w257) -> (w265:i16[])
            n207 = Insert Into Array(array=w259, index=w268, new element=w256) -> (w264:i16[])
          }
          frame True {
            n208 = call <vilib>:"Amplitude and Phase Spectrum.vi"("dt"=w270, "Signal (V)"=w276) -> ("Amp Spectrum Mag (Vrms)"=→"?":dbl[])  [unwired: 1 in, 2 out]
            n209 = call <vilib>:"Amplitude and Phase Spectrum.vi"("dt"=w270, "Signal (V)"=w275) -> ("Amp Spectrum Mag (Vrms)"=→"?":dbl[])  [unwired: 1 in, 2 out]
            n210 = call <vilib>:"Amplitude and Phase Spectrum.vi"("dt"=w270, "Signal (V)"=w277) -> ("Amp Spectrum Mag (Vrms)"=→"?":dbl[])  [unwired: 1 in, 2 out]
            n211 = call <vilib>:"Amplitude and Phase Spectrum.vi"("dt"=w270, "Signal (V)"=w278) -> ("Amp Spectrum Mag (Vrms)"=→"?":dbl[])  [unwired: 1 in, 2 out]
          }
        }
        n212 = Add(x=w252, y=w234) -> (x+y=w253:i32)
        "收包" <- w253
        n213 = Tick Count (ms)() -> (millisecond timer value=w244:u32)
        n214 = Subtract(x=w244, y=w245) -> (x-y=w243:u32)
        n215 = Subtract(x=w253, y=w252) -> (x-y=w251:i32)
        n216 = Add(x=w251, y=w250) -> (x+y=w246:i32)
        n217 = Add(x=w240, y=w243) -> (x+y=w241:u32)
        n218 = Greater Or Equal?(x=w246, y=1000000) -> (x >= y?=w248:bool)
        n219 = Or(x=w220, y=w219) -> (x .or. y?=w218:bool)
        n220 = case shown="真" w248 {
          tunnel: [w628 0] -> w247
          tunnel: w246 -> [w628 w631]
          tunnel: [w627 u32 0] -> w242
          tunnel: w241 -> [w627 w632]
          frame False {
          }
          frame True {
            n221 = Divide(x=w631, y=w632) -> (x/y=→"KB/s":dbl)
          }
        }
      }
    }
  }
